vi "ConvertImageUnit.vi"(10 "unit":T1=enum."counts", 11 "Images in Counts":dbl[][](array[numeric])) -> (1 "shot noise coefficient (sigma2)":dbl, 3 "converted image":dbl[][](array[numeric]))   [LabVIEW 2018]
uses:
  typedef/ImageUnit.ctl
  References.vi
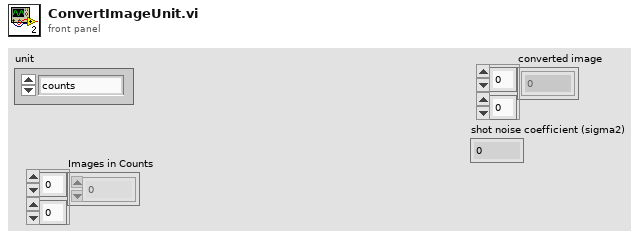
[diagram p1: front panel]
types:
  T1 = typedef "ImageUnit.ctl" = enum16{"Nphotons", "Efficiency", "I(uW/cm^2)", "I(nW/cm^2)", "Nelectrons", "I[W/cm^2]", "counts"}
  T2 = typedef "IMG_DATA_FORMAT.ctl" = enum16{"MONO8", "MONO16", "RGB24", "RGB32", "RGBPLANAR", "RAW8", "RAW16"}
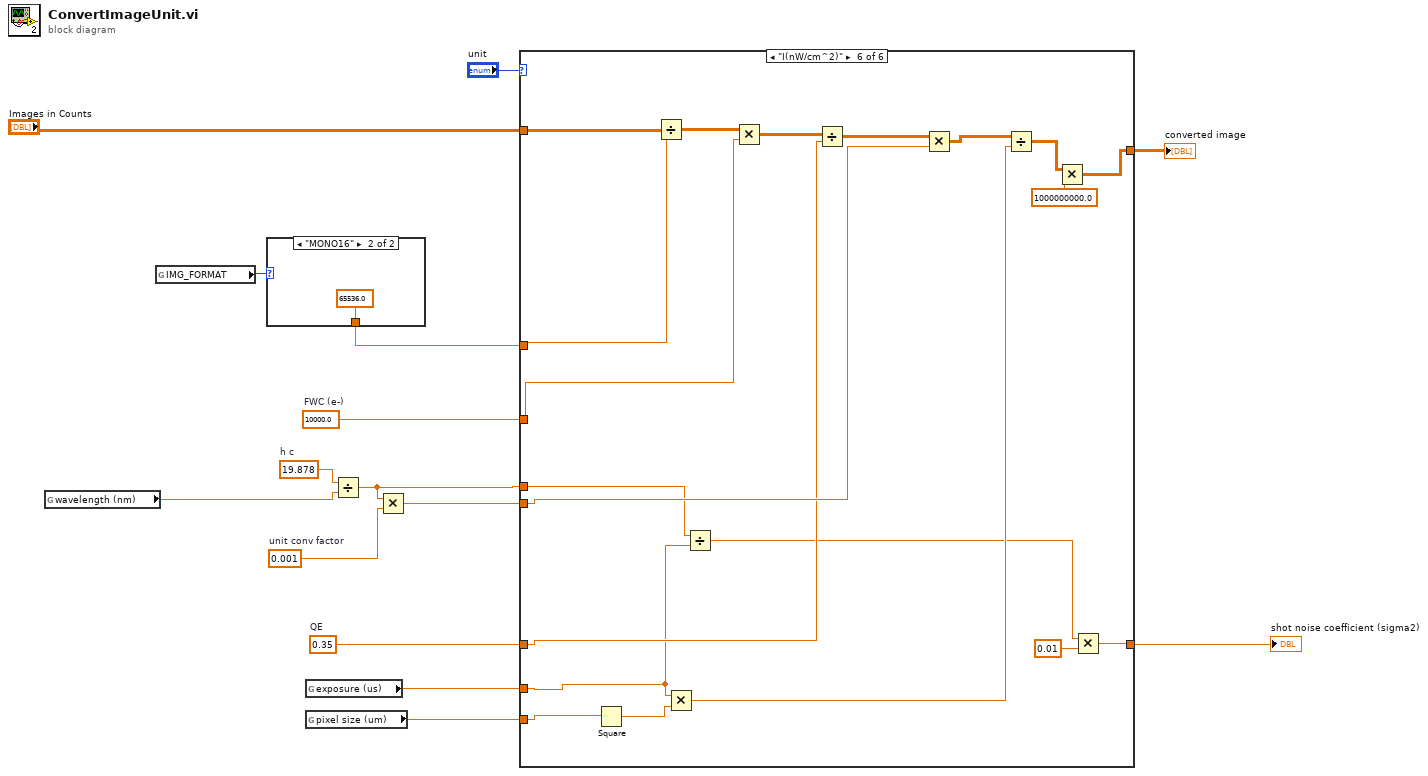
[diagram p0: block diagram]
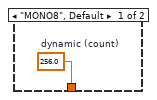
[diagram p2: hidden frame]
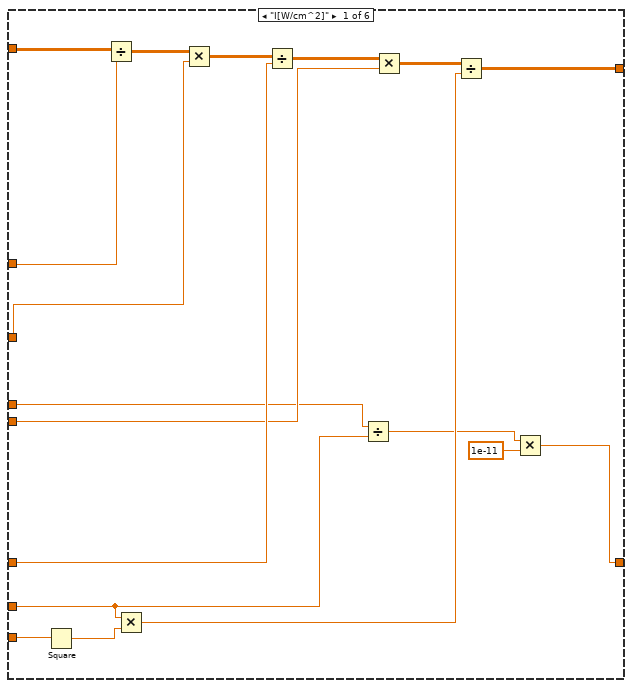
[diagram p3: hidden frame]
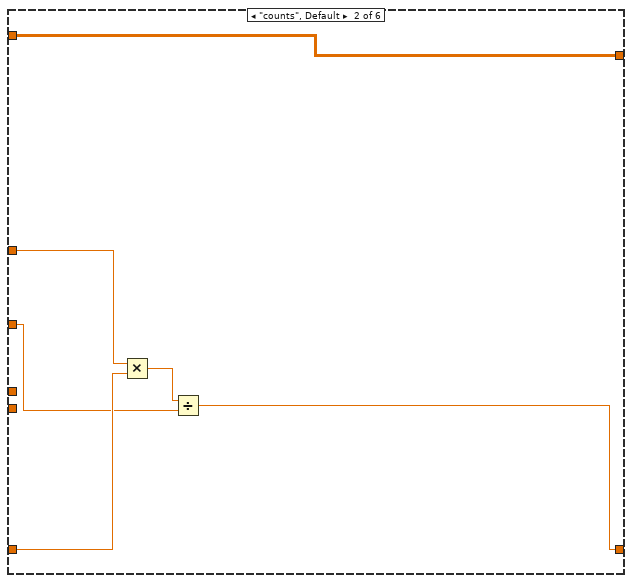
[diagram p4: hidden frame]
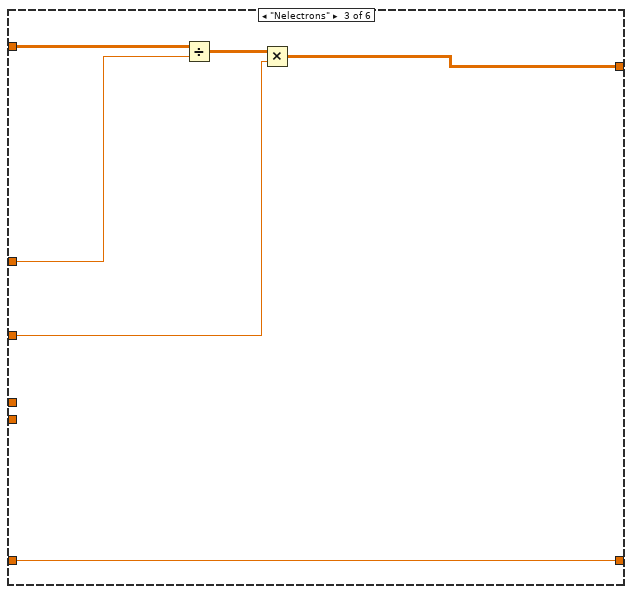
[diagram p5: hidden frame]
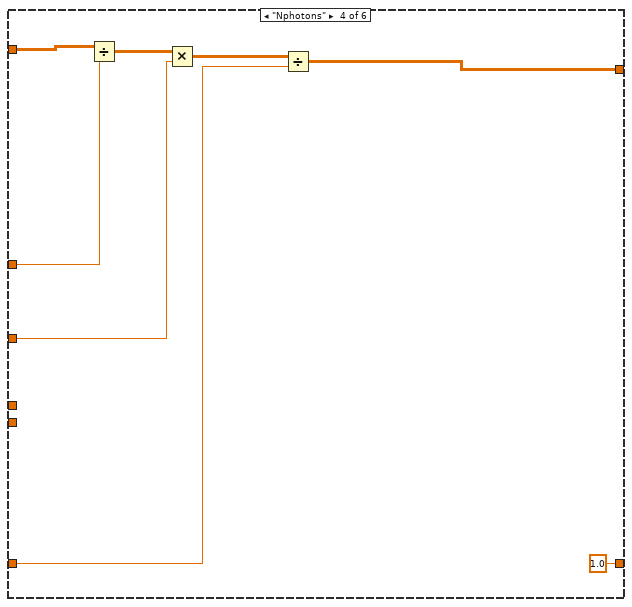
[diagram p6: hidden frame]
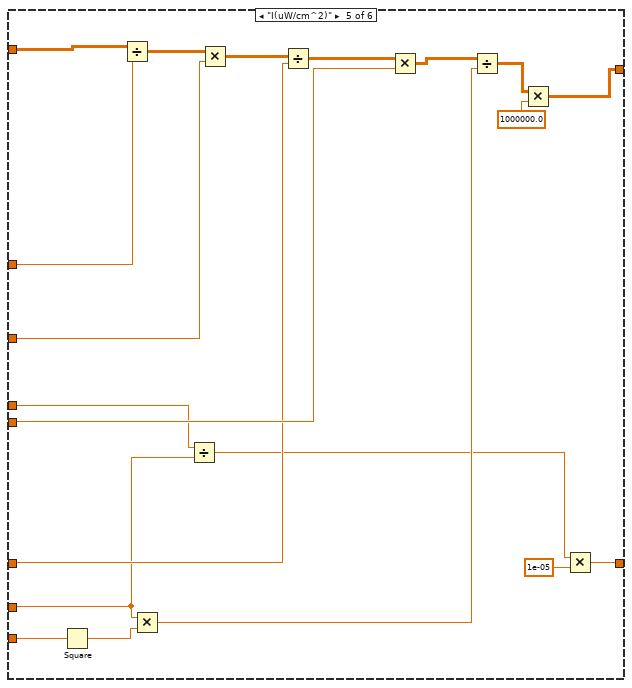
[diagram p7: hidden frame]
diagram:
  w6 = 0.001  # unit conv factor
  w8 = 19.878  # h c
  w12 = 0.35  # QE
  w13 = 10000.0  # FWC (e-)
  n1 = global read "References.vi" "wavelength (nm)"() -> (w7:dbl)
  n2 = global read "References.vi" "IMG_FORMAT"() -> (w10:T2)
  n3 = case shown="\"MONO16\"" w10 {
    tunnel: [w16 65536.0 ("dynamic (count)")] -> w9
    frame "MONO8", Default {
      w16 = 256.0  # dynamic (count)
    }
    frame "MONO16" {
    }
  }
  n4 = global read "References.vi" "exposure (us)"() -> (w11:dbl)
  n5 = global read "References.vi" "pixel size (um)"() -> (w4:dbl)
  n6 = Divide(x=w8, y=w7) -> (x/y=w1:dbl)
  n7 = Multiply(x=w1, y=w6) -> (x*y=w5:dbl)
  n8 = case shown="\"I(nW/cm^2)\"" "unit" {
    tunnel: [w29 w41 w45 w49 w61 w87] -> w15
    tunnel: "Images in Counts" -> [w34 w41 w47 w54 w69 w86]
    tunnel: w9 -> [w33 w39 w44 w53 w68 w85]
    tunnel: w13 -> [w32 w37 w43 w52 w67 w84]
    tunnel: w12 -> [w30 w40 w42 w50 w64 w82]
    tunnel: w11 -> [w21 _ _ _ w59 w77]
    tunnel: w5 -> [w26 _ _ _ w66 w83]
    tunnel: w4 -> [w25 _ _ _ w65 w81]
    tunnel: [w19 w36 w42 1.0 ("QE") w58 w79] -> w2
    tunnel: w1 -> [w22 _ _ _ w60 w78]
    frame "I[W/cm^2]" {
      n9 = Square(x=w25) -> (x^2=w24:dbl)
      n10 = Divide(x=w34, y=w33) -> (x/y=w35:dbl[][])
      n11 = Multiply(x=w21, y=w24) -> (x*y=w23:dbl)
      n12 = Multiply(x=w35, y=w32) -> (x*y=w31:dbl[][])
      n13 = Divide(x=w31, y=w30) -> (x/y=w28:dbl[][])
      n14 = Divide(x=w22, y=w21) -> (x/y=w20:dbl)
      n15 = Multiply(x=w28, y=w26) -> (x*y=w27:dbl[][])
      n16 = Divide(x=w27, y=w23) -> (x/y=w29:dbl[][])
      n17 = Multiply(x=w20, y=1e-11) -> (x*y=w19:dbl)
    }
    frame "counts", Default {
      n18 = Multiply(x=w39, y=w40) -> (x*y=w38:dbl)
      n19 = Divide(x=w38, y=w37) -> (x/y=w36:dbl)
    }
    frame "Nelectrons" {
      n20 = Divide(x=w47, y=w44) -> (x/y=w46:dbl[][])
      n21 = Multiply(x=w46, y=w43) -> (x*y=w45:dbl[][])
    }
    frame "Nphotons" {
      n22 = Divide(x=w54, y=w53) -> (x/y=w55:dbl[][])
      n23 = Multiply(x=w55, y=w52) -> (x*y=w51:dbl[][])
      n24 = Divide(x=w51, y=w50) -> (x/y=w49:dbl[][])
    }
    frame "I(uW/cm^2)" {
      n25 = Square(x=w65) -> (x^2=w71:dbl)
      n26 = Divide(x=w69, y=w68) -> (x/y=w75:dbl[][])
      n27 = Multiply(x=w59, y=w71) -> (x*y=w70:dbl)
      n28 = Divide(x=w60, y=w59) -> (x/y=w57:dbl)
      n29 = Multiply(x=w75, y=w67) -> (x*y=w74:dbl[][])
      n30 = Divide(x=w74, y=w64) -> (x/y=w73:dbl[][])
      n31 = Multiply(x=w73, y=w66) -> (x*y=w72:dbl[][])
      n32 = Divide(x=w72, y=w70) -> (x/y=w63:dbl[][])
      n33 = Multiply(x=w63, y=1000000.0) -> (x*y=w61:dbl[][])
      n34 = Multiply(x=w57, y=1e-05) -> (x*y=w58:dbl)
    }
    frame "I(nW/cm^2)" {
      n35 = Square(x=w81) -> (x^2=w91:dbl)
      n36 = Divide(x=w86, y=w85) -> (x/y=w95:dbl[][])
      n37 = Multiply(x=w77, y=w91) -> (x*y=w90:dbl)
      n38 = Divide(x=w78, y=w77) -> (x/y=w76:dbl)
      n39 = Multiply(x=w95, y=w84) -> (x*y=w94:dbl[][])
      n40 = Divide(x=w94, y=w82) -> (x/y=w93:dbl[][])
      n41 = Multiply(x=w93, y=w83) -> (x*y=w92:dbl[][])
      n42 = Divide(x=w92, y=w90) -> (x/y=w89:dbl[][])
      n43 = Multiply(x=w89, y=1000000000.0) -> (x*y=w87:dbl[][])
      n44 = Multiply(x=w76, y=0.01) -> (x*y=w79:dbl)
    }
  }
  "converted image" <- w15
  "shot noise coefficient (sigma2)" <- w2
